vi "Read ADC.vi"(8 "error in (no error)":errorcluster, 10 "ADC Channel Selection":T1=enum."Single Ended 0", 11 "ExplorerHatPro in":refnum<class "LINX-ExplorerHatPro.lvclass">) -> (0 "error out":errorcluster, 2 "ADC Volts":dbl, 3 "ExplorerHatPro out":refnum<class "LINX-ExplorerHatPro.lvclass">)   [LabVIEW 2020, in "LINX-ExplorerHatPro.lvclass"]
uses:
  LINX-ExplorerHatPro.lvclass
  LINX-ADS1015/LINX-ADS1X15.lvclass
  LINX-ADS1015/Channel Selection.ctl
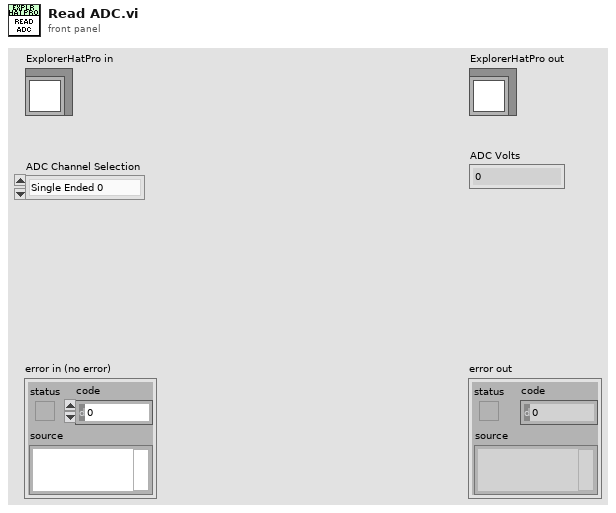
[diagram p1: front panel]
types:
  T1 = typedef "LINX-ADS1X15.lvclass/Channel Selection.ctl" = enum16{"Differential 0-1", "Differential 2-3", "Single Ended 0", "Single Ended 1", "Single Ended 2", "Single Ended 3"}
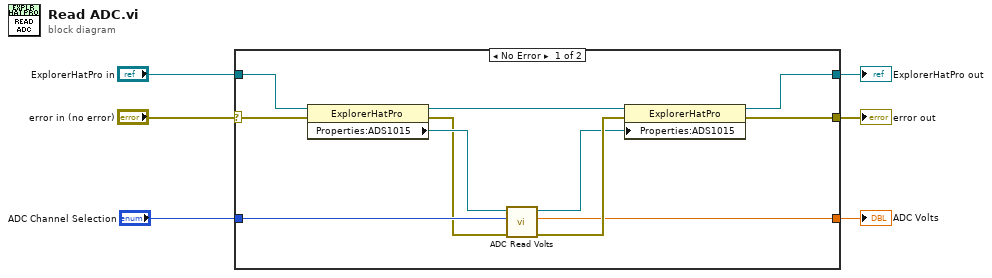
[diagram p0: block diagram]
diagram:
  n1 = case shown="No Error" "error in (no error)" {
    selector: "error in (no error)" -> [w14 w18]
    tunnel: [w7 w18] -> w5
    tunnel: [w11 w17] -> w3
    tunnel: "ExplorerHatPro in" -> [w16 w17]
    tunnel: "ADC Channel Selection" -> [w15 _]
    tunnel: [w8 _] -> w1
    frame No Error {
      n2 = property class="ExplorerHatPro"(reference=w16, error in=w14) -> (reference out=w11:refnum<class "LINX-ExplorerHatPro.lvclass">, error out=w12:errorcluster, "Properties:ADS1015"=w13:refnum<class "LINX-ADS1X15.lvclass">)
      n3 = call "ADC Read Volts.vi"("error in (no error)"=w12, "ADC Channel Selection"=w15, "LINX-ADS1X15 in"=w13) -> ("error out"=w10:errorcluster, "ADC Volts"=w8:dbl, "LINX-ADS1X15 out"=w9:refnum<class "LINX-ADS1X15.lvclass">)  [unwired: 6 in]
      n4 = property class="ExplorerHatPro"(reference=w11, error in=w10, "Properties:ADS1015"=w9) -> (error out=w7:errorcluster)  [unwired: 1 out]
    }
    frame Error {
    }
  }
  "error out" <- w5
  "ExplorerHatPro out" <- w3
  "ADC Volts" <- w1
